vi "Execute last step.vi"(8 "error in (no error)":errorcluster, 10 "Last Step done":bool, 11 "Car Wash Controller Actor in":refnum<class "Car Wash Controller Actor.lvclass">) -> (0 "error out":errorcluster, 3 "Car Wash Controller Actor out":refnum<class "Car Wash Controller Actor.lvclass">)   [LabVIEW 2019, in "Car Wash Controller Actor.lvlib" / "Car Wash Controller Actor.lvclass"]
uses:
  Car Wash Controller Actor.lvclass
  Car Wash Controller Actor.lvclass/Car Wash Controller Actor.ctl
  Simulated Wash Display Console Actor/Simulated Wash Display Console Actor Messages/Update Vehicle Out of Position Msg/Update Vehicle Out of Position Msg.lvclass/Update Vehicle Out of Position Msg.ctl
  <vilib>/ActorFramework/Message Enqueuer/Message Enqueuer.lvclass/Message Enqueuer.ctl
  Sim Entry Console Actor/Sim Entry Console Actor/Wash steps selection -Buttons.ctl
  Vehicle Position Simulation/Vehicle Position Simulation Messages/Update Vehicle Position Simulation Msg/Update Vehicle Position Simulation Msg.lvclass/Update Vehicle Position Simulation Msg.ctl
  Simulated Wash Display Console Actor/Simulated Wash Display Console Actor Messages/Update Car Wash Indicators Msg/Update Car Wash Indicators Msg.lvclass/Update Car Wash Indicators Msg.ctl
  <vilib>/ActorFramework/Message Enqueuer/Enqueue.vi
  Simulated Wash Display Console Actor/Simulated Wash Display Console Actor Messages/Update Vehicle Out of Position Msg/Update Vehicle Out of Position Msg.lvclass
  C:/Program Files (x86)/National Instruments/LabVIEW 2019/vi.lib/ActorFramework/Message/Message.lvclass
  Vehicle Position Simulation/Vehicle Position Simulation Messages/Update Vehicle Position Simulation Msg/Update Vehicle Position Simulation Msg.lvclass
  Simulated Wash Display Console Actor/Simulated Wash Display Console Actor Messages/Update Car Wash Indicators Msg/Update Car Wash Indicators Msg.lvclass
  <vilib>/ActorFramework/Message Priority Queue/Priority Enqueue.vi
  Sim Entry Console Actor/Sim Entry Console Actor/Simulated Entry Console Actor.lvclass
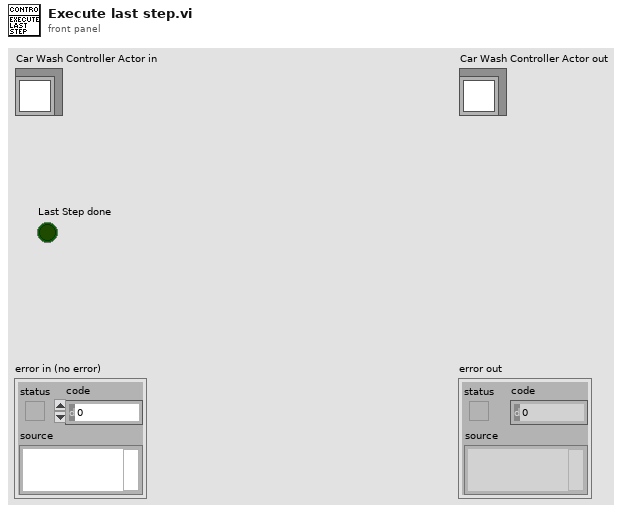
[diagram p1: front panel]
types:
  T1 = typedef "Simulated Entry Console Actor.lvlib/Simulated Entry Console Actor.lvclass/Wash steps selection -Buttons.ctl" = cluster{"Under Body Wash":bool, "Bug Remover":bool, "Pre-Soak":bool, "High Pressure Wash (default)":bool, "Low Pressure Wax":bool, "Spot Free Rinse":bool, "Tire Shine Foam":bool, "Air Dry":bool}
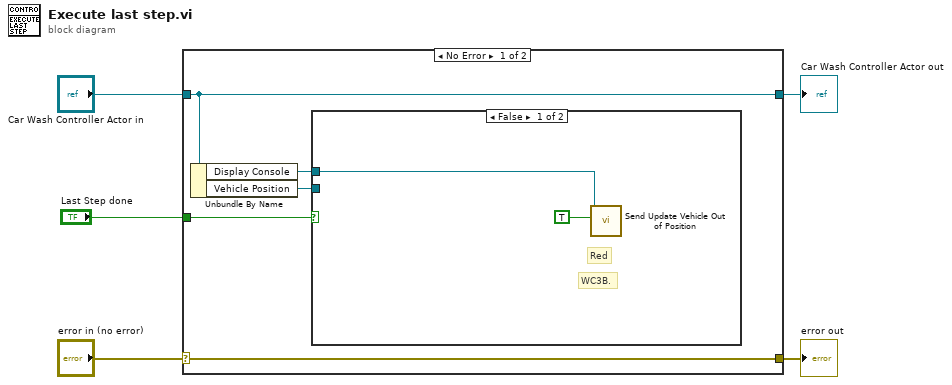
[diagram p0: block diagram]
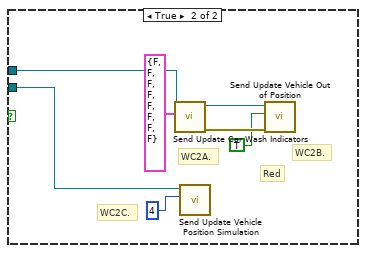
[diagram p2: hidden frame]
diagram:
  n1 = case shown="No Error" "error in (no error)" {
    selector: "error in (no error)" -> [w10 w21]
    tunnel: [w10 w21] -> w4
    tunnel: [w6 w20] -> w2
    tunnel: "Car Wash Controller Actor in" -> [w6 w20]
    tunnel: "Last Step done" -> [w9 _]
    frame No Error {
      n2 = Unbundle By Name(w6) -> ("Display Console"=w8:refnum<class "Message Enqueuer.lvclass">, "Vehicle Position"=w7:refnum<class "Message Enqueuer.lvclass">)
      n3 = case shown="False" w9 {
        tunnel: w8 -> [w11 w15]
        tunnel: w7 -> [_ w14]
        frame False {
          # "Red"
          # "WC3B."
          n4 = call "Send Update Vehicle Out of Position.vi"("Out of pos?"=TRUE, "Message Enqueuer"=w11) -> ()  [unwired: 8 in, 2 out]
        }
        frame True {
          # "WC2B."
          # "WC2C."
          # "Red"
          # "WC2A."
          n5 = call "Send Update Car Wash Indicators.vi"("Car Wash Indicators"=T1 {"Under Body Wash"=FALSE, "Bug Remover"=FALSE, "Pre-Soak"=FALSE, "High Pressure Wash (default)"=FALSE, "Low Pressure Wax"=FALSE, "Spot Free Rinse"=FALSE, "Tire Shine Foam"=FALSE, "Air Dry"=FALSE}, "Message Enqueuer"=w15) -> ("error out"=w18:errorcluster, "Message Enqueuer out"=w19:refnum<class "Message Enqueuer.lvclass">)  [unwired: 8 in]
          n6 = call "Send Update Vehicle Position Simulation.vi"("Vehicle Pos"=u32 4, "Message Enqueuer"=w14) -> ()  [unwired: 8 in, 2 out]
          n7 = call "Send Update Vehicle Out of Position.vi"("error in (no error)"=w18, "Out of pos?"=TRUE, "Message Enqueuer"=w19) -> ()  [unwired: 7 in, 2 out]
        }
      }
    }
    frame Error {
    }
  }
  "error out" <- w4
  "Car Wash Controller Actor out" <- w2
